vi "Close all.vi"() -> (0 "Errors":errorcluster[](array[cluster]))   [LabVIEW 2014]
uses:
  Coherent global.vi
panel:
  # "PN 04/11/2014"
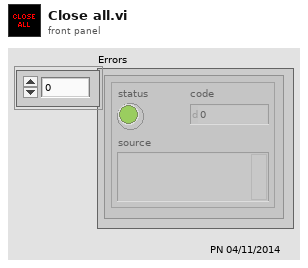
[diagram p1: front panel]
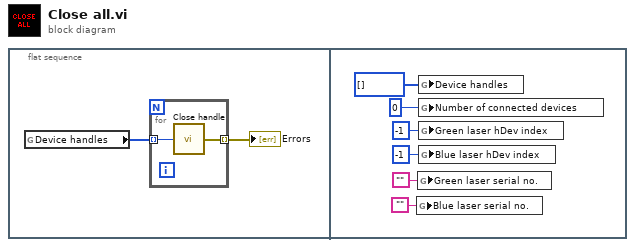
[diagram p0: block diagram]
diagram:
  n1 = flat-sequence {
    frame #0 {
      n2 = global read "Coherent global.vi" "Device handles"() -> (w2:u32[])
      n3 = for {
        tunnel: w2 -> [w4] mode=indexing
        tunnel: [w3] -> w1 mode=indexing
        n4 = call "Close handle.vi"("Device Handle"=w4) -> ("Error"=w3:errorcluster)
      }
      "Errors" <- w1
    }
    frame #1 {
      n5 = global write "Coherent global.vi" "Blue laser serial no."("" ("Blue laser serial no.")) -> ()
      n6 = global write "Coherent global.vi" "Green laser serial no."("" ("Green laser serial no.")) -> ()
      n7 = global write "Coherent global.vi" "Device handles"(u32[] [] ("Device handles")) -> ()
      n8 = global write "Coherent global.vi" "Number of connected devices"(u32 0 ("Number of connected devices")) -> ()
      n9 = global write "Coherent global.vi" "Green laser hDev index"(-1 ("Green laser hDev index")) -> ()
      n10 = global write "Coherent global.vi" "Blue laser hDev index"(-1 ("Blue laser hDev index")) -> ()
    }
  }
